vi "Default Instrument Setup.vi"(8 "error in (no error) 2":errorcluster, 11 "VISA resource name 2":refnum<visa-resource-name>) -> (0 "error out":errorcluster, 3 "VISA resource name out":refnum<visa-resource-name>)   [LabVIEW 2016, in "Tektronix AFG 1000 Series.lvlib"]
doc: "Sends a default command string to the instrument whenever a new VISA session is opened, or the instrument is reset. This VI is intended to be used as a subVI for the <B>Initialize</B> and <B> Reset</B> VI's. Altering this VI could cause these two VI's to operate incorrectly."
uses:
  Tektronix AFG 1000 Series.lvlib
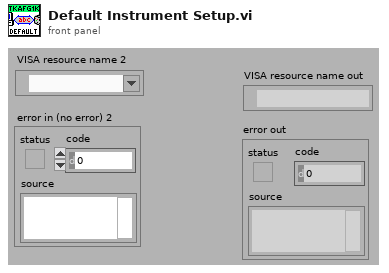
[diagram p1: front panel]
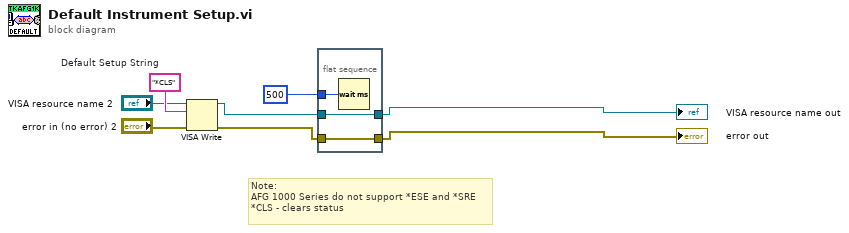
[diagram p0: block diagram]
diagram:
  w7 = "*CLS"  # Default Setup String
  # "Note:\nAFG 1000 Series do not support *ESE and *SRE\n*CLS - clears status"
  n1 = VISA Write(VISA resource name="VISA resource name 2", write buffer=w7, error in (no error)="error in (no error) 2") -> (VISA resource name out=w4:refnum<visa-resource-name>, error out=w3:errorcluster)  [unwired: 1 out]
  n2 = flat-sequence {
    tunnel: w3 -> [w10]
    tunnel: w4 -> [w11]
    tunnel: [w11] -> w2
    tunnel: [w10] -> w1
    tunnel: u32 500 ("milliseconds to wait") -> [w9]
    frame #0 {
      n3 = Wait (ms)(milliseconds to wait=w9) -> ()  [unwired: 1 out]
    }
  }
  "error out" <- w1
  "VISA resource name out" <- w2
